vi "Start.vi"(8 "error in (no error)":errorcluster, 11 "Task in":refnum<class "PWM.lvclass">) -> (0 "error out":errorcluster, 3 "Task out":refnum<class "PWM.lvclass">)   [LabVIEW 2009, in "MicroDAQ.lvlib" / "PWM.lvclass"]
uses:
  <instrlib>/MicroDAQ/Channel/PWM/PWM.lvclass
  <instrlib>/MicroDAQ/Channel/PWM/PWM.lvclass/PWM.ctl
  <instrlib>/MicroDAQ/Mlink library wraper/mlink.lvlib
  <instrlib>/MicroDAQ/Channel/Channel.lvclass
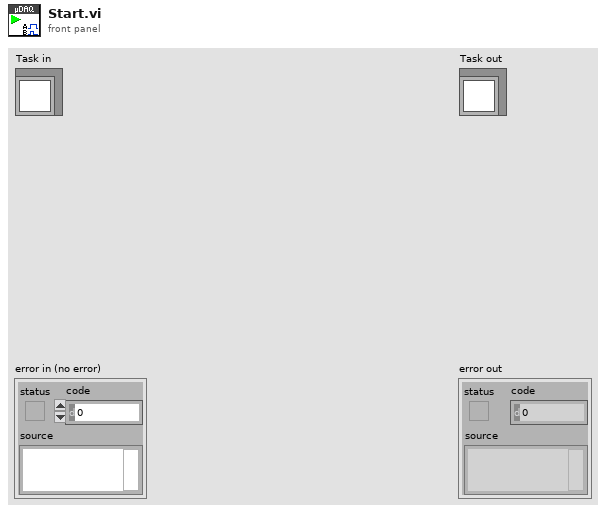
[diagram p1: front panel]
types:
  T1 = typedef "MicroDAQ.lvlib/PWM channel.ctl" = enum8{"None", "PWM1", "PWM2", "PWM3"}
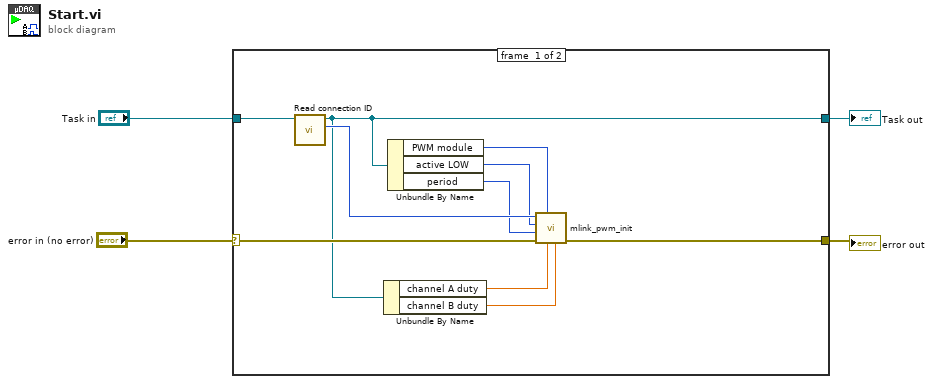
[diagram p0: block diagram]
diagram:
  n1 = case shown="No Error" "error in (no error)" {
    selector: "error in (no error)" -> [w14 w15]
    tunnel: [w13 w15] -> w3
    tunnel: "Task in" -> [w12 w16]
    tunnel: [w7 w16] -> w1
    frame #0 {
      n2 = call <instrlib>:"Read connection ID.vi"("Task in"=w12) -> ("connection ID"=w11:i32, "Task out"=w7:refnum<class "PWM.lvclass">)  [unwired: 9 in]
      n3 = Unbundle By Name(w7) -> ("channel A duty"=w6:sgl, "channel B duty"=w5:sgl)
      n4 = Unbundle By Name(w7) -> ("PWM module"=w10:T1, "active LOW"=w9:u8, "period"=w8:u32)
      n5 = call <instrlib>:"mlink_pwm_init.vi"("channel B duty"=w5, "channel A duty"=w6, "PWM module"=w10, "error in (no error)"=w14, "period"=w8, "active LOW"=w9, "connection ID"=w11) -> ("error out"=w13:errorcluster)  [unwired: 3 in, 1 out]
    }
    frame #1 {
    }
  }
  "error out" <- w3
  "Task out" <- w1
